vi "Helper.vi"   [LabVIEW 2015, in "Main Controller Actor.lvclass"]
uses:
  Main Controller Actor.lvclass
  Process.vi
types:
  T1 = enum32{"Invalid", "Standard", "Closed", "Hidden", "Minimized", "Maximized"}
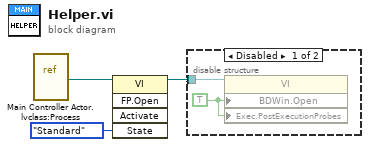
[diagram p0: block diagram]
diagram:
  n1 = vi-ref "Main Controller Actor.lvclass:Process.vi"() -> (w3:refnum<vi>)
  n2 = invoke class="VI" method="FP.Open"(reference=w3, "State"=T1."Standard") -> (reference out=w1:refnum<vi>)  [unwired: 3 in, 4 out]
  n3 = disable-structure shown="Disabled" {
    disable-tunnel: w1 -> [w5 _]
    frame Disabled {
      w4 = TRUE ("Block Diagram Window:Open")
      n4 = property class="VI"(reference=w5, "BDWin.Open"=w4, "Exec.PostExecutionProbes"=w4) -> ()  [unwired: 1 in, 2 out]
    }
    frame Enabled {
    }
  }
